vi "prepareStiffnessBaseline.vi"(6 "Distance to Plate Measured":dbl[unit]=1.0 min=1.0 max=300.0 format="%.1f", 8 "error in (no error)":errorcluster, 9 "Encoder Position":dbl[unit], 10 "Force Measured":T1 min=-888.0 max=888.0 format="%.2f", 11 "StiffnessMonitor in":refnum<class "StiffnessMonitor.lvclass">) -> (0 "error out":errorcluster, 3 "StiffnessMonitor out":refnum<class "StiffnessMonitor.lvclass">)   [LabVIEW 2015, in "StiffnessMonitor.lvclass"]
uses:
  StiffnessMonitor.lvclass
  Typedefs/ForceDemand.ctl
  StiffnessMonitor.lvclass/StiffnessMonitor.ctl
  Typedefs/M1M3SSSTypedefs.lvlib
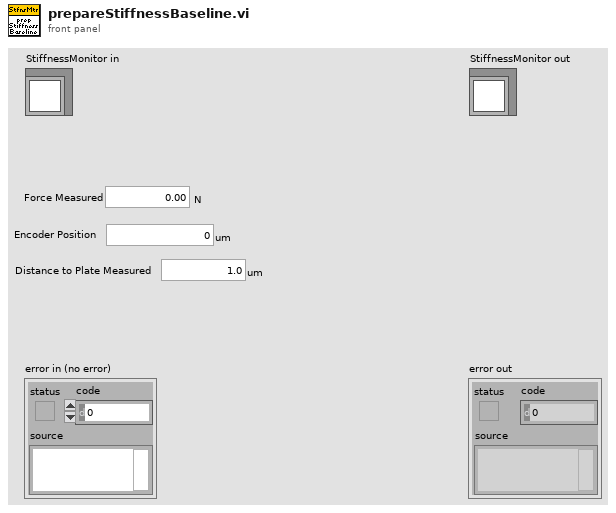
[diagram p1: front panel]
types:
  T1 = typedef "M1M3SSSTypedefs.lvlib/ForceDemand.ctl" = dbl[unit]
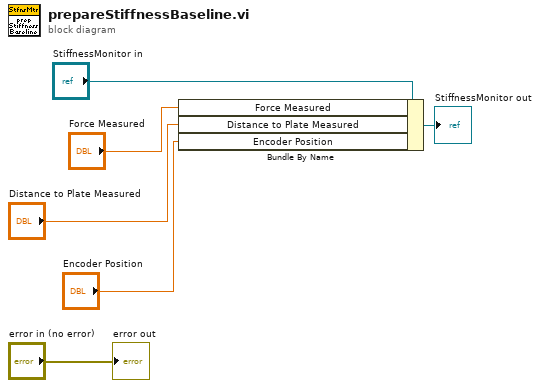
[diagram p0: block diagram]
diagram:
  n1 = Bundle By Name(cluster="StiffnessMonitor in", "Force Measured"="Force Measured", "Distance to Plate Measured"="Distance to Plate Measured", "Encoder Position"="Encoder Position") -> (→"StiffnessMonitor out":refnum<class "StiffnessMonitor.lvclass">)
  "error out" <- "error in (no error)"
